vi "VI Server Control.vi"(0 "VI Server Control":T1={"VI name"="", "Control"=[], "Value"=[], "Boolean?"=[], "Control to End"="", "Condition"=enum."within xxx% of target value", "xxx%"=0.0, "Target Value"=0.0, "Timeout (sec)"=120.0, "wait (sec)"=120.0, "check every (s)"=120.0, "Boolean indi"=FALSE} {"Boolean?" min=0.0 max=1.0 step=1.0 format="%#_1g"}) -> ()   [LabVIEW 2025]
doc: "Author: Scott Hannahs <sth@magnet.fsu.edu>\n\nThis software is licensed for use under the “MIT License\"\nCopyright (c) 2025 Scott Hannahs, sth@sth@magnet.sthnet.net\n\nPermission is hereby granted, free of charge, to any person obtaining a copy of this software and associated documentation files (the \"Software\"), to deal in the Software without restriction, including without limitation the rights to use, copy, modify, merge, publish, distribute, sublicense, and/or sell copies of the Software, and to permit persons to whom the Software is furnished to do so, subject to the following conditions: The above copyright notice and this permission notice shall be included in all copies or substantial portions of the Software.\n\nTHE SOFTWARE IS PROVIDED \"AS IS\", WITHOUT WARRANTY OF ANY KIND, EXPRESS OR IMPLIED, INCLUDING BUT NOT LIMITED TO THE WARRANTIES OF MERCHANTABILITY, FITNESS FOR A PARTICULAR PURPOSE AND NONINFRINGEMENT. IN NO EVENT SHALL THE AUTHORS OR COPYRIGHT HOLDERS BE LIABLE FOR ANY CLAIM, DAMAGES OR OTHER LIABILITY, WHETHER IN AN ACTION OF CONTRACT, TORT OR OTHERWISE, ARISING FROM, OUT OF OR IN CONNECTION WITH THE SOFTWARE OR THE USE OR OTHER DEALINGS IN THE SOFTWARE."
uses:
  Units/VI Server Control N1/VI Server Control.ctl
panel:
  out "initial value":dbl
  out "error out":errorcluster
  # "0"
  # "1"
  # "2"
  # "3"
  # "4"
  # "5"
  # "6"
  # "7"
  # "8"
  # "9"
  # "Finish if"
  # "is"
  # "and also finish the whole thing if time elapses"
  # "or longer."
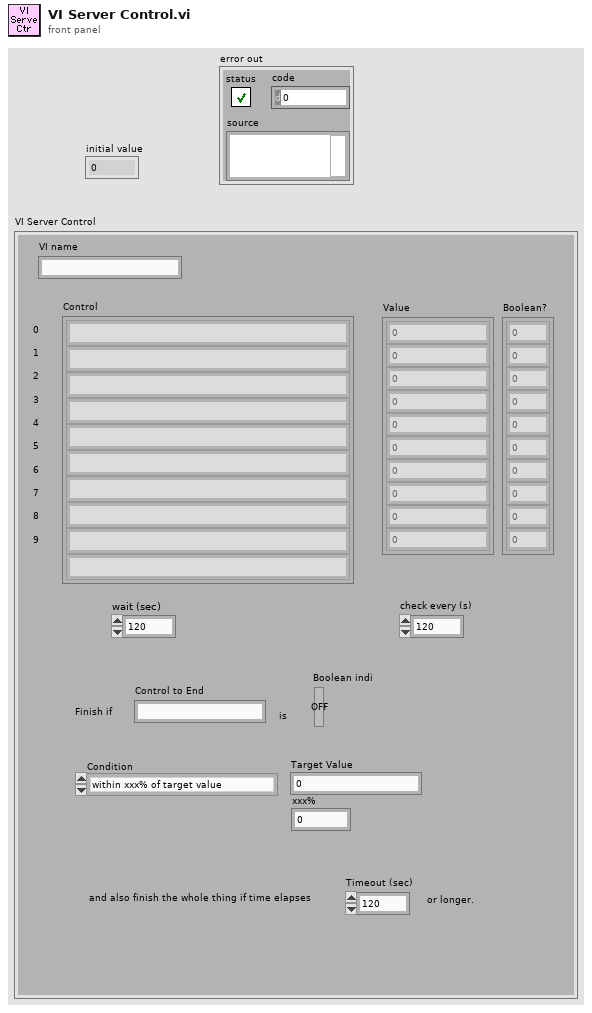
[diagram p1: front panel]
types:
  T1 = typedef "VI Server Control.ctl" = cluster{"VI name":string, "Control":string[], "Value":dbl[], "Boolean?":dbl[], "Control to End":string, "Condition":enum16{"within xxx% of target value", "<= target value", ">= target value", "= target value"}, "xxx%":dbl, "Target Value":dbl, "Timeout (sec)":dbl, "wait (sec)":dbl, "check every (s)":dbl, "Boolean indi":bool}
  T2 = enum16{"within xxx% of target value", "<= target value", ">= target value", "= target value"}
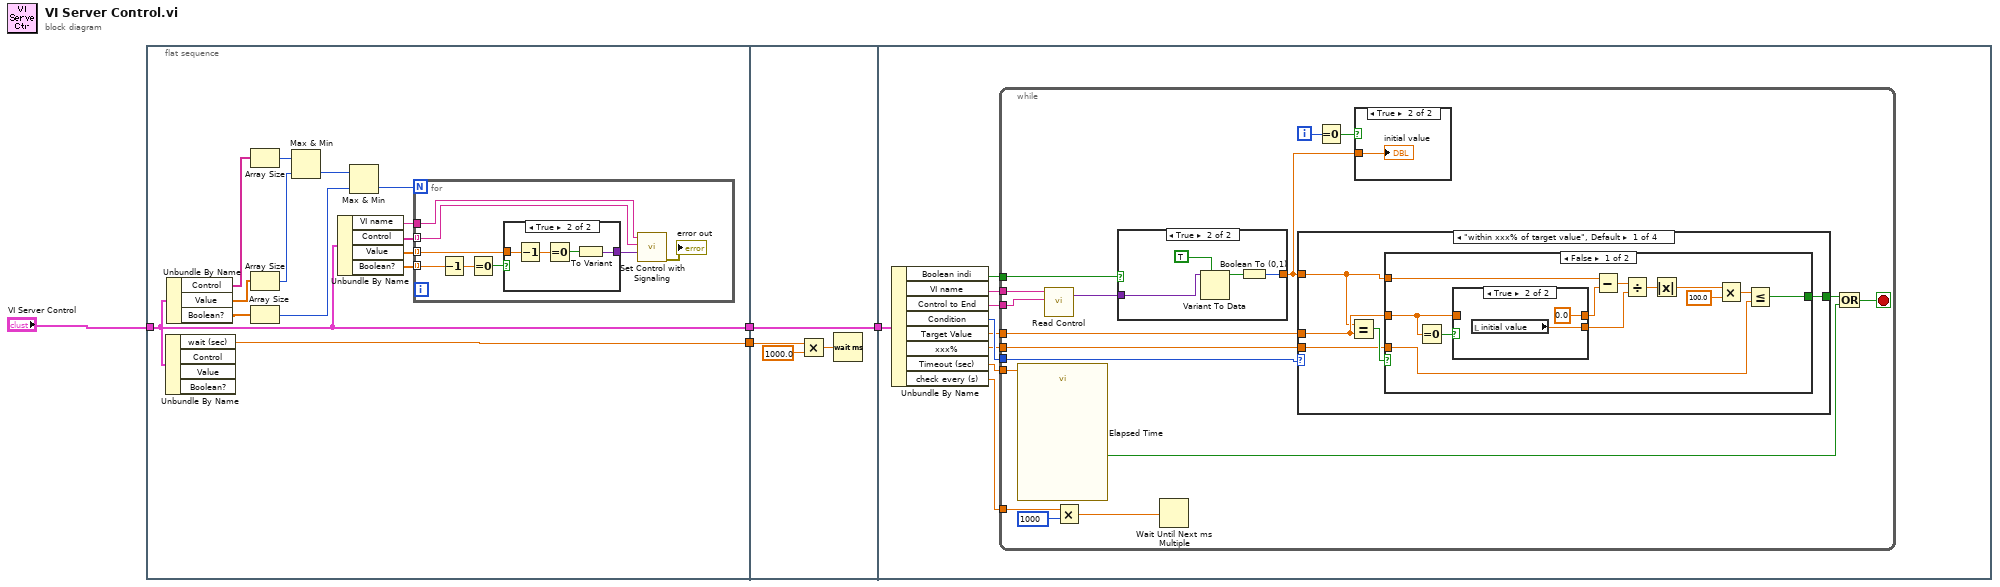
[diagram p0: block diagram]
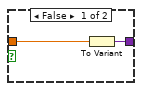
[diagram p2: hidden frame]
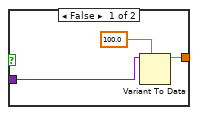
[diagram p4: hidden frame]
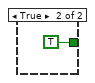
[diagram p6: hidden frame]
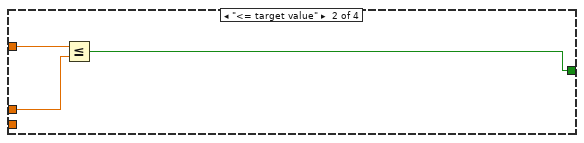
[diagram p7: hidden frame]
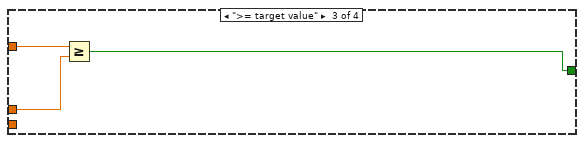
[diagram p8: hidden frame]
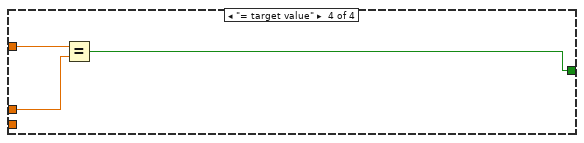
[diagram p9: hidden frame]
diagram:
  n1 = flat-sequence {
    tunnel: "VI Server Control" -> [w5]
    tunnel: [w6] -> w3
    tunnel: [w5] -> w1
    tunnel: w3 -> [w35]
    tunnel: [w33] -> w2
    tunnel: w1 -> [w33]
    tunnel: w2 -> [w45]
    frame #0 {
      n2 = Unbundle By Name(w5) -> ("wait (sec)"=w6:dbl)  [unwired: 3 out]
      n3 = Unbundle By Name(w5) -> ("Control"=w18:string[], "Value"=w17:dbl[], "Boolean?"=w11:dbl[])
      n4 = Array Size(array=w18) -> (size(s)=w16:i32)
      n5 = Array Size(array=w17) -> (size(s)=w15:i32)
      n6 = Array Size(array=w11) -> (size(s)=w13:i32)
      n7 = Max & Min(x=w16, y=w15) -> (min(x,y)=w14:i32)  [unwired: 1 out]
      n8 = Unbundle By Name(w5) -> ("VI name"=w8:string, "Control"=w7:string[], "Value"=w9:dbl[], "Boolean?"=w10:dbl[])
      n9 = Max & Min(x=w14, y=w13) -> (min(x,y)=w12:i32)  [unwired: 1 out]
      n10 = for {
        N: w12 -> [_]
        tunnel: w10 -> [w26] mode=indexing
        tunnel: w9 -> [w23] mode=indexing
        tunnel: w8 -> [w22]
        tunnel: w7 -> [w20] mode=indexing
        n11 = Decrement(x=w26) -> (x-1=w25:dbl)
        n12 = Equal To 0?(x=w25) -> (x = 0?=w24:bool)
        n13 = case shown="True" w24 {
          tunnel: w23 -> [w27 w31]
          tunnel: [w28 w30] -> w21
          frame False {
            n14 = To Variant(anything=w27) -> (Variant=w28:variant)
          }
          frame True {
            n15 = Decrement(x=w31) -> (x-1=w32:dbl)
            n16 = Equal To 0?(x=w32) -> (x = 0?=w29:bool)
            n17 = To Variant(anything=w29) -> (Variant=w30:variant)
          }
        }
        n18 = call "Set Control with Signaling.vi"("Value"=w21, "Control Name"=w20, "VI Name"=w22) -> ("error out"=→"error out":errorcluster)  [unwired: 8 in]
      }
    }
    frame #1 {
      n19 = Multiply(x=w35, y=1000.0) -> (x*y=w34:dbl)
      n20 = Wait (ms)(milliseconds to wait=w34) -> ()  [unwired: 1 out]
    }
    frame #2 {
      n21 = Unbundle By Name(w45) -> ("Boolean indi"=w37:bool, "VI name"=w44:string, "Control to End"=w43:string, "Condition"=w42:T2, "Target Value"=w41:dbl, "xxx%"=w40:dbl, "Timeout (sec)"=w39:dbl, "check every (s)"=w38:dbl)
      n22 = while {
        tunnel: w44 -> [w62]
        tunnel: w43 -> [w61]
        tunnel: w42 -> [w59]
        tunnel: w41 -> [w58]
        tunnel: w40 -> [w57]
        tunnel: w39 -> [w54]
        tunnel: w38 -> [w51]
        tunnel: w37 -> [w49]
        i -> [w48]
        stop <- w55 stop-if-true
        n23 = call "Elapsed Time"("Time Target (s)"=w54) -> ("Time has Elapsed"=w53:bool)  [unwired: 11 in, 7 out]
        n24 = call "Read Control.vi"("VI Name"=w62, "Control Name"=w61) -> ("Value"=w60:variant)  [unwired: 3 in, 1 out]
        n25 = Multiply(x=w51, y=1000) -> (x*y=w50:dbl)
        n26 = case shown="True" w49 {
          tunnel: w60 -> [w65 w70]
          tunnel: [w64 w67] -> w46
          frame False {
            n27 = Variant To Data(type=100.0 ("y"), Variant=w65) -> (data=w64:dbl)  [unwired: 1 in, 1 out]
          }
          frame True {
            n28 = Variant To Data(type=TRUE, Variant=w70) -> (data=w68:bool)  [unwired: 1 in, 1 out]
            n29 = Boolean To (0,1)(Boolean=w68) -> (0, 1=w67:i16)
          }
        }
        n30 = Wait Until Next ms Multiple(millisecond multiple=w50) -> ()  [unwired: 1 out]
        n31 = case shown="\"within xxx% of target value\", Default" w59 {
          tunnel: w58 -> [w73 w92 w95 w98]
          tunnel: [w74 w94 w97 w100] -> w56
          tunnel: w57 -> [w72 _ _ _]
          tunnel: w46 -> [w71 w93 w96 w99]
          frame "within xxx% of target value", Default {
            n32 = Equal?(x=w71, y=w73) -> (x = y?=w75:bool)
            n33 = case shown="False" w75 {
              tunnel: [w79 TRUE] -> w74
              tunnel: w73 -> [w82 _]
              tunnel: w72 -> [w83 _]
              tunnel: w71 -> [w76 _]
              frame False {
                n34 = Equal To 0?(x=w82) -> (x = 0?=w87:bool)
                n35 = case shown="True" w87 {
                  tunnel: [w88 0.0 ("Target Value")] -> w78
                  tunnel: w82 -> [w88 _]
                  tunnel: [w88 w89] -> w77
                  frame False {
                  }
                  frame True {
                    n36 = local read "initial value"() -> (w89:dbl)
                  }
                }
                n37 = Subtract(x=w76, y=w78) -> (x-y=w80:dbl)
                n38 = Divide(x=w80, y=w77) -> (x/y=w81:dbl)
                n39 = Absolute Value(x=w81) -> (abs(x)=w84:dbl)
                n40 = Multiply(x=w84, y=100.0) -> (x*y=w85:dbl)
                n41 = Less Or Equal?(x=w85, y=w83) -> (x <= y?=w79:bool)
              }
              frame True {
              }
            }
          }
          frame "<= target value" {
            n42 = Less Or Equal?(x=w93, y=w92) -> (x <= y?=w94:bool)
          }
          frame ">= target value" {
            n43 = Greater Or Equal?(x=w96, y=w95) -> (x >= y?=w97:bool)
          }
          frame "= target value" {
            n44 = Equal?(x=w99, y=w98) -> (x = y?=w100:bool)
          }
        }
        n45 = Equal To 0?(x=w48) -> (x = 0?=w47:bool)
        n46 = case shown="True" w47 {
          tunnel: w46 -> [_ w63]
          frame False {
          }
          frame True {
            "initial value" <- w63
          }
        }
        n47 = Or(x=w56, y=w53) -> (x .or. y?=w55:bool)
      }
    }
  }
